vi "Motor_generatemotion.vi"(1 "Conversion\n (steps/mm)":dbl[](array[numeric])=[12500.0, 31496.063, 31496.063, 31496.063] format="%#_13g", 2 "Distance  (mm)":dbl[](array[numeric])=[0.0, 0.0, 0.0, 0.0] format="%#_13g") -> (0 "Movement String":string)   [LabVIEW 2018]
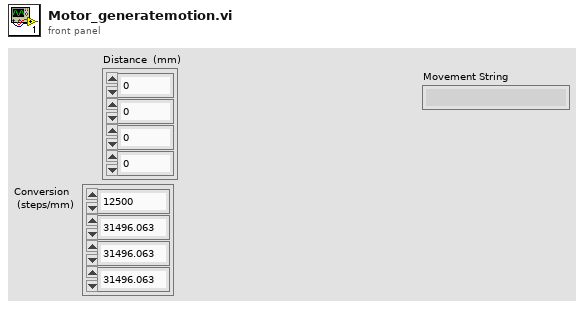
[diagram p1: front panel]
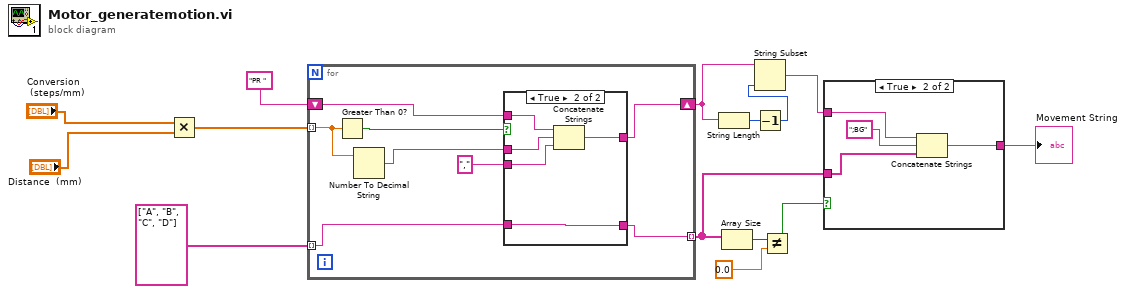
[diagram p0: block diagram]
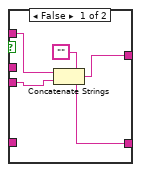
[diagram p3: hidden frame]
diagram:
  n1 = Multiply(x="Conversion\n (steps/mm)", y="Distance  (mm)") -> (x*y=w12:dbl[])
  n2 = for {
    tunnel: w12 -> [w16] mode=indexing
    tunnel: string[] ["A", "B", "C", "D"] -> [w22] mode=indexing
    tunnel: [w19] -> w7 mode=indexing
    shift-right: [w18] -> w4
    shift-left: "PR " ("string") -> [w17]
    n3 = Greater Than 0?(x=w16) -> (x > 0?=w15:bool)
    n4 = Number To Decimal String(number=w16) -> (decimal integer string=w21:string)  [unwired: 1 in]
    n5 = case shown="True" w15 {
      tunnel: w22 -> [_ w31]
      tunnel: ["" w31] -> w19
      tunnel: w21 -> [_ w30]
      tunnel: [w23 w29] -> w18
      tunnel: "," -> [w24 w28]
      tunnel: w17 -> [w25 w27]
      frame False {
        n6 = Concatenate Strings(w25, w24) -> (w23:string)
      }
      frame True {
        n7 = Concatenate Strings(w27, w30, w28) -> (w29:string)
      }
    }
  }
  n8 = String Length(string=w4) -> (length=w3:i32)
  n9 = Array Size(array=w7) -> (size(s)=w9:i32)
  n10 = Decrement(x=w3) -> (x-1=w2:i32)
  n11 = String Subset(string=w4, length (rest)=w2) -> (substring=w1:string)  [unwired: 1 in]
  n12 = Not Equal?(x=w9, y=0.0) -> (x != y?=w10:bool)
  n13 = case shown="True" w10 {
    tunnel: w7 -> [_ w35]
    tunnel: w1 -> [w32 w36]
    tunnel: [w32 w33] -> w6
    frame False {
    }
    frame True {
      n14 = Concatenate Strings(w36, ";BG" ("string"), w35) -> (w33:string)
    }
  }
  "Movement String" <- w6
